vi "Clear Type Descriptor Map.vi"(8 "error in (no error)":errorcluster, 11 "TwinCAT ADS in":refnum<class "TwinCAT ADS.lvclass">) -> (0 "error out":errorcluster, 2 "[TypeName:Descriptor Pair]":T1(array[cluster]), 3 "TwinCAT ADS out":refnum<class "TwinCAT ADS.lvclass">)   [LabVIEW 2018, in "TwinCAT ADS.lvclass"]
uses:
  TwinCAT ADS.lvclass
  TwinCAT ADS.lvclass/TwinCAT ADS.ctl
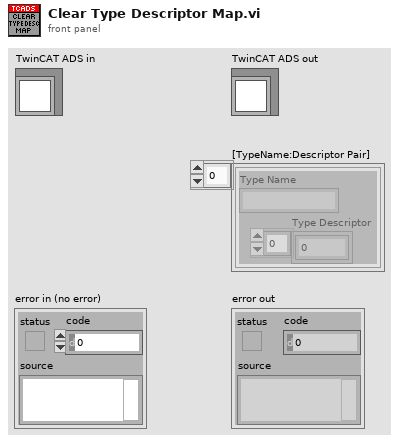
[diagram p1: front panel]
types:
  T1 = cluster{"Type Name":string, "Type Descriptor":i16[]}[]
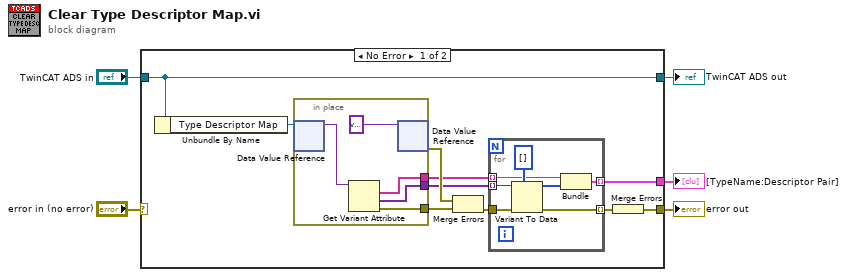
[diagram p0: block diagram]
diagram:
  n1 = case shown="No Error" "error in (no error)" {
    selector: "error in (no error)" -> [_ w28]
    tunnel: "TwinCAT ADS in" -> [w13 w29]
    tunnel: [w13 w29] -> w4
    tunnel: [w6 w28] -> w2
    tunnel: [w9 _] -> w1
    frame No Error {
      n2 = Unbundle By Name(w13) -> ("Type Descriptor Map"=w14:refnum<data-value>)
      n3 = in-place {
        in-place-border: [w25] -> w10
        in-place-border: [w24] -> w11
        in-place-border: [w23] -> w8
        n4 = in-place-dvr #1(w14) -> (w27:variant)  [unwired: 1 out]
        n5 = Get Variant Attribute(Variant=w27) -> (names=w25:string[], values=w24:variant[], error out=w23:errorcluster)  [unwired: 3 in, 1 out]
        n6 = in-place-dvr #1(variant ("data value")) -> (w15:errorcluster)  [unwired: 1 out]
      }
      n7 = Merge Errors(w15, w8) -> (w12:errorcluster)
      n8 = for {
        tunnel: w12 -> [w21]
        tunnel: w11 -> [w20] mode=indexing
        tunnel: w10 -> [w18] mode=indexing
        tunnel: [w17] -> w9 mode=indexing
        tunnel: [w16] -> w7 mode=indexing
        n9 = Variant To Data(error in=w21, type=i16[] [] ("Type Descriptor"), Variant=w20) -> (data=w19:i16[], error out=w16:errorcluster)
        n10 = Bundle(w18, "Type Descriptor"=w19) -> (w17:cluster{string, "Type Descriptor":i16[]})  [unwired: 1 in]
      }
      n11 = Merge Errors(w7) -> (w6:errorcluster)
    }
    frame Error {
    }
  }
  "error out" <- w2
  "TwinCAT ADS out" <- w4
  "[TypeName:Descriptor Pair]" <- w1
